vi "stat.vi"(8 "error in (no error)":errorcluster, 11 "Signals":dynamicdata(waveform)) -> (0 "error out":errorcluster, 1 "stDev":dbl, 2 "mean":dbl, 4 "min":dbl, 5 "max":dbl)   [LabVIEW 2020, in "main.lvlib"]
uses:
  main.lvlib
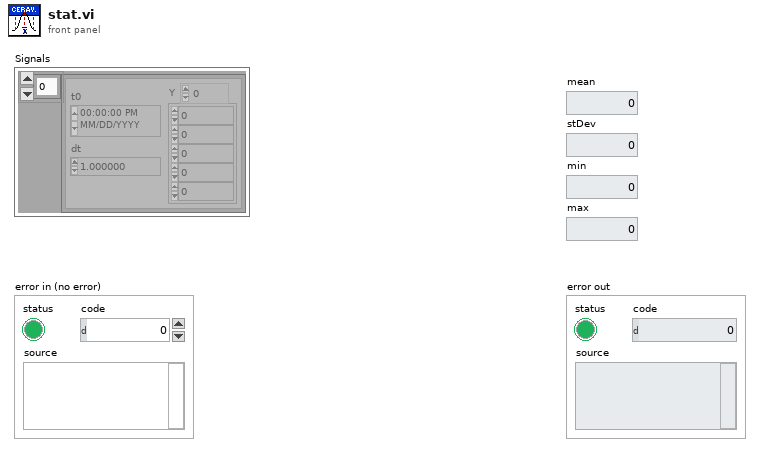
[diagram p1: front panel]
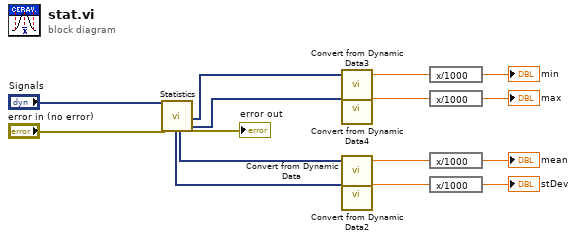
[diagram p0: block diagram]
diagram:
  n1 = call "Statistics"("Signals"="Signals", "error in (no error)"="error in (no error)") -> ("Standard Dev"=w11:dynamicdata, "Arithmetic Mean"=w12:dynamicdata, "Minimum"=w6:dynamicdata, "Maximum"=w5:dynamicdata, "error out"=→"error out":errorcluster)  [unwired: 21 in]
  n2 = call "Convert from Dynamic Data3"("Dynamic Data Type"=w6) -> ("Scalar"=w8:dbl)  [unwired: 3 in]
  n3 = call "Convert from Dynamic Data4"("Dynamic Data Type"=w5) -> ("Scalar"=w7:dbl)  [unwired: 3 in]
  n4 = call "Convert from Dynamic Data"("Dynamic Data Type"=w12) -> ("Scalar"=w9:dbl)  [unwired: 3 in]
  n5 = call "Convert from Dynamic Data2"("Dynamic Data Type"=w11) -> ("Scalar"=w10:dbl)  [unwired: 3 in]
  n6 = expression code="x/1000"(w8) -> (→"min":dbl)
  n7 = expression code="x/1000"(w7) -> (→"max":dbl)
  n8 = expression code="x/1000"(w9) -> (→"mean":dbl)
  n9 = expression code="x/1000"(w10) -> (→"stDev":dbl)
